vi "GEA2 Script_Progress.vi"(0 "Total iterations":i32, 9 "Current iteration":i32) -> (4 "Completion percent":dbl, 10 "Current test":string)   [LabVIEW 2023]
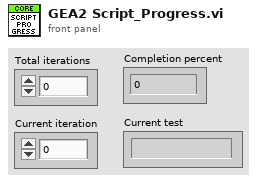
[diagram p1: front panel]
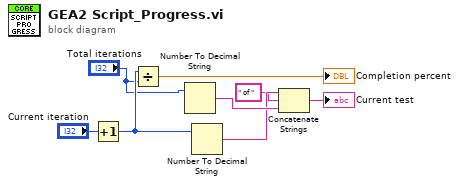
[diagram p0: block diagram]
diagram:
  n1 = Increment(x="Current iteration") -> (x+1=w8:i32)
  n2 = Divide(x=w8, y="Total iterations") -> (x/y=→"Completion percent":dbl)
  n3 = Number To Decimal String(number="Total iterations") -> (decimal integer string=w6:string)  [unwired: 1 in]
  n4 = Number To Decimal String(number=w8) -> (decimal integer string=w5:string)  [unwired: 1 in]
  n5 = Concatenate Strings(w5, " of " ("string"), w6) -> (→"Current test":string)
